vi "Filter Errors.vi"(11 "error in (no error)":errorcluster) -> (3 "error out":errorcluster)   [LabVIEW 2021]
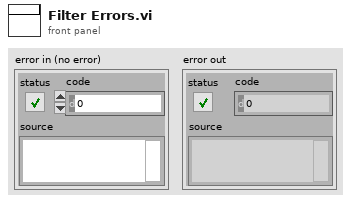
[diagram p1: front panel]
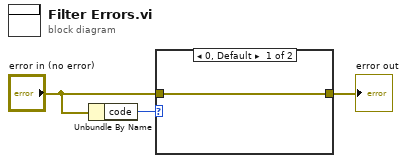
[diagram p0: block diagram]
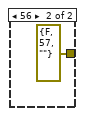
[diagram p2: hidden frame]
diagram:
  n1 = Unbundle By Name("error in (no error)") -> ("code"=w3:i32)
  n2 = case shown="0, Default" w3 {
    tunnel: "error in (no error)" -> [w4 _]
    tunnel: [w4 errorcluster {"status"=FALSE, "code"=57, "source"=""} ("error in (no error)")] -> w1
    frame 0, Default {
    }
    frame 56 {
    }
  }
  "error out" <- w1
